vi "high pass filter.vi"() -> ()   [LabVIEW 2010]
uses:
  <vilib>/Utility/file.llb/Write To Spreadsheet File (I64).vi
panel:
  out "x-y":u16=178
  out "Current Aquisiton":u16[](graph)=[1897, 1897, 1897, 1893, 1891, 1889, 1889, 1886, 1885, 1882, 1880, 1875, 1870, 1866, 1863, 1859, 1857, 1852, 1848, 1844, 1839, 1835, 1832, 1829, 1827, 1825, 1821, 1811, 1806, 1801, 1798, 1795, 1794, 1791, 1788, 1786, 1781, 1776, 1771, 1768, 1764, 1762, 1758, 1755, 1751, 1746, 1744, 1742, 1740, 1737, 1737, 1735, 1734, 1733, 1730, 1727, 1728, 1726, 1727, 1726, 1727, 1727, 1726, 1725, 1723, 1728, 1728, 1730, 1730, 1731, 1731, 1732, 1733, 1736, 1738, 1741, 1744, 1745, 1749, 1750, 1752, 1755, 1760, 1764, 1769, 1773, 1776, 1779, 1782, 1786, 1788, 1793, 1797, 1813, 1822, 1826, 1830, 1833, 1837, 1841, 1846, 1850, 1855, 1857, 1861, 1864, 1867, 1871, 1876, 1877, 1882, 1884, 1886, 1888, 1889, 1892, 1893, 1894, 1897, 1898, 1897, 1897, 1897, 1899, 1898, 1900, 1900, 1900, 1898, 1897, 1896, 1895, 1897, 1896, 1894, 1894, 1892, 1889, 1885, 1883, 1880, 1878, 1874, 1873, 1869, 1864, 1858, 1854, 1850, 1846, 1843, 1840, 1837, 1833, 1829, 1826, 1824, 1818, 1810, 1806, 1803, 1800, 1797, 1793, 1790, 1786, 1783, 1781, 1777, 1772, 1769, 1764, 1759, 1757, 1754, 1751, 1749, 1748, 1742, 1740, 1737, 1733, 1733, 1734, 1732, 1731, 1729, 1729, 1726, 1726, 1725, 1726, 1726, 1726, 1728, 1727, 1729, 1726, 1727, 1729, 1733, 1732, 1734, 1736, 1736, 1737, 1739, 1740, 1746, 1749, 1752, 1755, 1758, 1760, 1764, 1767, 1772, 1777, 1781, 1785, 1787, 1789, 1792, 1796, 1813, 1822, 1828, 1832, 1834, 1838, 1841, 1845, 1850, 1854, 1859, 1864, 1866, 1869, 1872, 1874, 1876, 1881, 1886, 1888, 1890, 1890, 1893, 1892, 1895, 1896, 1897, 1899, 1900, 1899, 1898, 1897, 1898, 1899, 1898, 1898, 1900, 1899, 1896, 1894, 1894, 1893, 1891, 1890, 1890, 1887, 1884, 1880, 1877, 1872, 1870, 1867, 1865, 1859, 1855, 1850, 1846, 1842, 1838, 1835, 1834, 1830, 1827, 1824, 1816, 1808, 1804, 1802, 1800, 1797, 1794, 1790, 1786, 1781, 1778, 1775, 1773, 1769, 1766, 1761, 1757, 1753, 1750, 1746, 1745, 1743, 1742, 1738, 1736, 1732, 1730, 1730, 1731, 1729, 1729, 1727, 1726, 1727, 1725, 1726, 1726, 1728, 1730, 1728, 1727, 1728, 1729, 1730, 1732, 1736, 1736, 1736, 1737, 1740, 1741, 1744, 1748, 1751, 1754, 1759, 1761, 1764, 1768, 1772, 1777, 1781, 1786, 1789, 1791, 1793, 1798, 1814, 1822, 1827, 1833, 1836, 1839, 1842, 1846, 1850, 1854, 1858, 1862, 1867, 1869, 1873, 1875, 1877, 1882, 1885, 1888, 1889, 1892, 1891, 1894, 1893, 1896, 1897, 1899, 1899, 1899, 1899, 1898, 1898, 1897, 1898, 1899, 1898, 1899, 1897, 1896, 1894, 1893, 1893, 1892, 1890, 1886, 1883, 1880, 1877, 1872, 1870, 1867, 1863, 1861, 1855, 1850, 1845, 1841, 1838, 1836, 1832, 1830, 1826, 1824, 1814, 1807, 1804, 1802, 1799, 1797, 1794, 1790, 1785, 1781, 1778, 1775, 1773, 1769, 1765, 1760, 1754, 1750, 1750, 1746, 1746, 1742, 1741, 1738, 1733, 1733, 1733, 1731, 1730, 1731, 1730, 1726, 1725, 1726, 1726, 1726, 1727, 1728, 1728, 1729, 1727, 1728, 1728, 1730, 1733, 1734, 1736, 1736, 1738, 1739, 1742, 1746, 1748, 1752, 1756, 1759, 1762, 1765, 1768, 1773, 1777, 1782, 1785, 1788, 1791, 1793, 1801, 1815, 1824, 1829, 1833, 1837, 1839, 1842, 1846, 1850, 1854, 1860, 1864, 1867, 1870, 1872, 1875, 1877, 1881, 1885, 1888, 1889, 1891, 1891, 1893, 1895, 1897, 1898, 1900, 1901, 1898, 1897, 1896, 1898, 1899, 1899, 1900, 1898, 1896, 1897, 1895, 1893, 1893, 1892, 1890, 1889, 1886, 1882, 1880, 1876, 1873, 1870, 1867, 1864, 1859, 1854, 1849, 1844, 1841, 1838, 1835, 1833, 1829, 1826, 1823, 1814, 1807, 1803, 1801, 1799, 1796, 1794, 1789, 1785, 1781, 1778, 1776, 1772, 1768, 1764, 1759, 1756, 1753, 1749, 1747, 1745, 1743, 1741, 1736, 1734, 1733, 1731, 1731, 1730, 1729, 1727, 1728, 1726, 1724, 1726, 1726, 1728, 1728, 1727, 1729, 1729, 1728, 1728, 1730, 1734, 1733, 1736, 1737, 1738, 1741, 1743, 1745, 1749, 1753, 1757, 1759, 1762, 1764, 1769, 1774, 1778, 1782, 1786, 1789, 1791, 1793, 1803, 1817, 1824, 1830, 1833, 1836, 1839, 1842, 1845, 1851, 1855, 1860, 1864, 1867, 1871, 1872, 1875, 1880, 1882, 1886, 1887, 1888, 1891, 1891, 1892, 1894, 1895, 1897, 1899, 1899, 1899, 1897, 1898, 1897, 1898, 1897, 1899, 1898, 1897, 1894, 1895, 1892, 1891, 1893, 1890, 1890, 1887, 1882, 1879, 1874, 1872, 1869, 1866, 1863, 1859, 1854, 1849, 1844, 1841, 1837, 1834, 1832, 1829, 1826, 1823, 1813, 1806, 1802, 1801, 1798, 1797, 1792, 1788, 1785, 1780, 1777, 1774, 1771, 1769, 1763, 1759, 1755, 1750, 1748, 1745, 1746, 1742, 1741, 1739, 1734, 1734, 1731, 1730, 1731, 1731, 1728, 1726, 1726, 1727, 1725, 1726, 1726, 1727, 1730, 1729, 1730, 1728, 1730, 1730, 1733, 1735, 1736, 1739, 1740, 1740, 1742, 1745, 1747, 1754, 1758, 1761, 1763, 1766, 1769, 1772, 1778, 1782, 1786, 1789, 1792, 1794, 1805, 1817, 1824, 1829, 1834, 1838, 1841, 1843, 1846, 1851, 1855, 1859, 1865, 1868, 1871, 1874, 1876, 1880, 1881, 1886, 1888, 1890, 1891, 1893, 1893, 1894, 1896, 1896, 1897, 1899, 1899, 1899, 1897, 1897, 1898, 1901, 1899, 1900, 1898, 1897, 1895, 1894, 1892, 1890, 1890, 1889, 1886, 1882, 1880, 1875, 1871, 1867, 1865, 1862, 1858, 1853, 1849, 1844, 1840, 1837, 1834, 1832, 1829, 1826, 1824, 1812, 1806, 1802, 1800, 1798, 1796, 1793, 1789, 1784, 1781, 1777, 1774, 1771, 1767, 1763, 1760, 1755, 1751, 1746, 1746, 1744, 1742, 1740, 1740, 1736, 1732, 1730, 1730, 1730, 1730, 1729, 1730, 1727, 1726, 1726, 1725, 1727, 1728, 1728, 1730, 1730, 1728, 1730, 1730, 1733, 1735, 1737, 1739, 1739, 1741, 1743, 1745, 1750, 1752, 1757, 1760, 1764, 1766, 1770, 1774, 1778, 1782, 1787, 1790, 1793, 1795, 1807, 1818, 1824, 1829, 1833, 1838, 1842, 1845, 1848, 1851, 1855, 1860, 1864, 1870, 1873, 1876, 1877, 1879, 1882, 1884, 1888, 1892, 1893, 1893, 1893, 1894, 1895, 1897, 1897, 1899, 1900, 1900, 1898, 1899, 1898, 1896, 1897, 1898, 1898, 1898, 1896, 1894, 1891, 1890, 1888, 1889, 1886, 1884, 1880, 1876, 1870, 1867, 1863, 1860, 1857, 1854, 1848, 1845, 1840, 1835, 1833, 1830, 1828, 1826, 1823, 1813, 1806, 1801, 1799, 1797, 1795, 1792, 1789, 1786, 1781, 1776, 1773, 1769, 1766, 1763, 1759, 1757, 1751, 1748, 1743, 1742, 1741, 1741, 1738, 1736, 1734, 1731, 1730, 1730, 1727, 1729, 1729, 1728, 1726, 1728, 1725, 1725, 1726, 1730, 1728, 1730, 1731, 1730, 1730, 1731, 1734, 1736, 1738, 1742, 1743, 1744, 1746, 1749, 1753, 1756, 1761, 1765]
  in  "Auto Save Data":bool=TRUE
  in  "Data File path Ending":string=".dat"
  out "Previous Aquisition":u16[](graph)=[1899, 1898, 1899, 1897, 1897, 1897, 1899, 1900, 1898, 1900, 1898, 1897, 1900, 1898, 1898, 1898, 1897, 1898, 1900, 1898, 1901, 1896, 1899, 1899, 1896, 1899, 1900, 1897, 1901, 1898, 1897, 1898, 1897, 1899, 1900, 1896, 1898, 1897, 1899, 1898, 1897, 1899, 1899, 1898, 1900, 1897, 1899, 1898, 1897, 1899, 1899, 1897, 1899, 1898, 1899, 1899, 1896, 1899, 1897, 1898, 1900, 1898, 1899, 1896, 1898, 1898, 1898, 1897, 1899, 1898, 1900, 1898, 1897, 1899, 1897, 1898, 1899, 1897, 1899, 1898, 1898, 1899, 1898, 1898, 1898, 1897, 1897, 1898, 1899, 1899, 1897, 1901, 1898, 1898, 1900, 1897, 1899, 1900, 1896, 1898, 1898, 1898, 1900, 1898, 1898, 1901, 1896, 1899, 1899, 1897, 1900, 1897, 1898, 1899, 1897, 1899, 1897, 1897, 1900, 1897, 1899, 1899, 1897, 1900, 1898, 1898, 1898, 1897, 1898, 1899, 1897, 1899, 1898, 1897, 1899, 1895, 1900, 1900, 1899, 1900, 1897, 1897, 1899, 1896, 1898, 1898, 1896, 1898, 1897, 1897, 1898, 1896, 1898, 1898, 1898, 1899, 1896, 1898, 1898, 1897, 1898, 1897, 1899, 1901, 1898, 1898, 1899, 1896, 1900, 1898, 1897, 1900, 1899, 1897, 1900, 1898, 1900, 1898, 1899, 1900, 1898, 1900, 1899, 1898, 1898, 1897, 1898, 1899, 1897, 1900, 1898, 1897, 1900, 1897, 1897, 1898, 1896, 1899, 1898, 1897, 1901, 1897, 1898, 1900, 1898, 1898, 1899, 1898, 1901, 1896, 1898, 1898, 1897, 1901, 1898, 1898, 1898, 1898, 1898, 1898, 1897, 1900, 1898, 1898, 1899, 1897, 1899, 1898, 1897, 1898, 1899, 1898, 1899, 1897, 1899, 1898, 1898, 1898, 1897, 1898, 1899, 1897, 1899, 1899, 1900, 1900, 1897, 1899, 1898, 1898, 1899, 1899, 1898, 1899, 1898, 1899, 1900, 1897, 1900, 1898, 1898, 1899, 1896, 1899, 1899, 1897, 1899, 1897, 1898, 1899, 1898, 1898, 1898, 1899, 1899, 1896, 1897, 1899, 1897, 1900, 1899, 1899, 1899, 1897, 1898, 1899, 1897, 1899, 1898, 1898, 1900, 1896, 1899, 1898, 1898, 1900, 1898, 1899, 1900, 1897, 1899, 1898, 1898, 1898, 1899, 1898, 1900, 1898, 1900, 1899, 1897, 1899, 1897, 1900, 1899, 1897, 1899, 1898, 1897, 1900, 1897, 1897, 1898, 1896, 1900, 1899, 1899, 1901, 1898, 1899, 1900, 1897, 1899, 1898, 1898, 1899, 1898, 1899, 1900, 1897, 1900, 1897, 1897, 1899, 1897, 1900, 1899, 1896, 1900, 1897, 1898, 1900, 1896, 1898, 1898, 1897, 1899, 1896, 1898, 1900, 1896, 1900, 1899, 1897, 1901, 1899, 1899, 1899, 1899, 1899, 1898, 1897, 1900, 1898, 1899, 1899, 1897, 1900, 1898, 1898, 1898, 1896, 1898, 1900, 1897, 1898, 1898, 1898, 1901, 1896, 1900, 1898, 1898, 1899, 1898, 1898, 1898, 1898, 1898, 1898, 1897, 1899, 1897, 1897, 1899, 1898, 1899, 1897, 1897, 1898, 1896, 1899, 1899, 1897, 1899, 1898, 1897, 1901, 1897, 1899, 1898, 1897, 1899, 1898, 1896, 1899, 1896, 1898, 1898, 1896, 1899, 1897, 1899, 1899, 1898, 1897, 1899, 1896, 1899, 1897, 1898, 1898, 1897, 1900, 1898, 1897, 1898, 1898, 1899, 1898, 1897, 1899, 1897, 1898, 1897, 1899, 1898, 1897, 1896, 1899, 1899, 1897, 1899, 1897, 1898, 1897, 1897, 1899, 1897, 1898, 1900, 1894, 1899, 1898, 1898, 1898, 1897, 1899, 1899, 1897, 1898, 1898, 1899, 1899, 1897, 1898, 1898, 1897, 1899, 1898, 1896, 1898, 1897, 1898, 1900, 1898, 1898, 1898, 1897, 1898, 1896, 1898, 1898, 1896, 1900, 1897, 1898, 1900, 1897, 1899, 1899, 1899, 1899, 1895, 1898, 1898, 1897, 1898, 1897, 1898, 1898, 1895, 1897, 1898, 1897, 1897, 1897, 1897, 1899, 1895, 1897, 1897, 1897, 1899, 1898, 1897, 1900, 1896, 1898, 1898, 1896, 1899, 1898, 1896, 1898, 1897, 1898, 1897, 1897, 1899, 1896, 1898, 1898, 1896, 1897, 1897, 1897, 1899, 1896, 1897, 1898, 1896, 1898, 1897, 1897, 1898, 1897, 1898, 1897, 1897, 1898, 1898, 1898, 1898, 1896, 1897, 1897, 1896, 1899, 1897, 1897, 1898, 1896, 1899, 1897, 1896, 1899, 1898, 1896, 1897, 1897, 1897, 1896, 1896, 1900, 1896, 1898, 1898, 1896, 1899, 1896, 1897, 1899, 1895, 1899, 1898, 1896, 1898, 1898, 1895, 1899, 1896, 1898, 1897, 1894, 1897, 1897, 1895, 1898, 1896, 1896, 1899, 1896, 1898, 1898, 1897, 1898, 1899, 1897, 1896, 1896, 1898, 1897, 1897, 1898, 1897, 1899, 1896, 1896, 1898, 1896, 1897, 1897, 1897, 1898, 1896, 1896, 1898, 1896, 1897, 1898, 1897, 1897, 1896, 1897, 1898, 1896, 1897, 1897, 1896, 1899, 1896, 1896, 1898, 1895, 1898, 1897, 1893, 1898, 1895, 1897, 1897, 1894, 1898, 1896, 1896, 1896, 1895, 1897, 1897, 1896, 1898, 1896, 1895, 1897, 1894, 1897, 1898, 1896, 1897, 1897, 1896, 1897, 1897, 1898, 1896, 1897, 1897, 1896, 1897, 1897, 1895, 1897, 1897, 1897, 1897, 1896, 1896, 1897, 1896, 1897, 1898, 1896, 1897, 1895, 1897, 1897, 1894, 1896, 1897, 1896, 1896, 1894, 1896, 1897, 1894, 1897, 1896, 1896, 1897, 1896, 1896, 1895, 1895, 1897, 1897, 1895, 1897, 1896, 1897, 1897, 1895, 1897, 1896, 1896, 1897, 1895, 1897, 1897, 1895, 1897, 1895, 1896, 1894, 1894, 1896, 1897, 1894, 1897, 1893, 1895, 1898, 1894, 1896, 1894, 1894, 1897, 1895, 1897, 1898, 1894, 1897, 1897, 1894, 1897, 1895, 1894, 1895, 1895, 1897, 1896, 1896, 1897, 1894, 1897, 1897, 1894, 1898, 1894, 1896, 1897, 1893, 1897, 1897, 1894, 1898, 1895, 1894, 1897, 1895, 1897, 1895, 1893, 1897, 1894, 1895, 1896, 1895, 1897, 1895, 1895, 1897, 1895, 1895, 1897, 1895, 1897, 1894, 1895, 1895, 1893, 1896, 1894, 1894, 1897, 1894, 1894, 1896, 1893, 1897, 1897, 1894, 1897, 1894, 1895, 1896, 1895, 1896, 1896, 1893, 1897, 1894, 1895, 1896, 1893, 1897, 1893, 1894, 1897, 1894, 1895, 1895, 1892, 1895, 1894, 1893, 1896, 1894, 1895, 1896, 1894, 1894, 1896, 1894, 1895, 1894, 1894, 1894, 1894, 1895, 1894, 1896, 1895, 1893, 1895, 1895, 1893, 1895, 1894, 1894, 1896, 1894, 1896, 1894, 1894, 1895, 1894, 1893, 1896, 1893, 1895, 1894, 1894, 1894, 1894, 1895, 1895, 1893, 1895, 1893, 1894, 1895, 1894, 1896, 1895, 1893, 1894, 1894, 1895, 1894, 1893, 1895, 1895, 1892, 1895, 1891, 1895, 1896, 1891, 1896, 1893, 1893, 1896, 1893, 1894, 1893, 1894, 1894, 1894, 1894, 1894, 1892, 1895, 1894, 1893, 1895, 1893, 1893, 1896, 1893, 1895, 1894, 1891, 1895, 1892, 1893, 1895, 1892, 1894, 1894, 1894, 1894, 1894, 1893, 1894, 1893, 1893, 1894, 1891, 1893, 1893, 1894, 1895, 1892, 1895, 1895, 1894, 1896, 1891, 1894, 1894, 1894, 1893, 1894, 1893, 1894, 1893, 1894, 1893, 1891, 1893, 1892, 1893, 1894, 1892, 1893, 1892, 1892, 1893, 1892, 1893, 1894, 1891, 1894, 1893, 1892, 1893, 1891, 1893, 1893]
  in  "time format string (%c)":string="%Y-%m-%d %H-%M.%S"
  out "date/time string":string="2012-02-22 16-27.20"
  in  "InterChannel Delay":sgl=-1.0 format="%.2f"
  out "ErrMsg":string="No error has occurred"
  out "ErrCode":i32
  in  "BoardNum":u32
  in  "LowChan":i32
  in  "HighChan":i32
  in  "Options":i32
  in  "Range":i32(ring)=1 items=["Not Programmable"=0, "+- 20 V"=27, "+- 10 V"=1, "+- 5 V"=2, "+- 4 V"=28, "+- 2.5 V"=3, "+- 2 V"=29, "+- 1.67 V"=4, "+- 1.25 V"=5, "+- 1 V"=6, "+- .625 V"=7, "+- .5 V"=8, "+- .25 V"=30, "+- .2 V"=31, "+- .1 V"=9, "+- .05 V"=10, "+- .01 V"=11, "+- .005 V"=12, "0 - 10 V"=13, "0 - 5 V"=14, "0 - 4 V"=36, "0 - 2.5 V"=15, "0 - 2 V"=16, "0 - 1.67 V"=17, "0 - 1.25 V"=18, "0 - 1 V"=19, "0 - .5 V"=32, "0 - .25 V"=33, "0 - .2 V"=34, "0 - .1 V"=20, "0 - .02 V"=35, "0 - .01 V"=21, "4 - 20 mA"=22, "2 - 10 mA"=23, "1 - 5 mA"=24, ".5 - 2.5 mA"=25, "0 - 20 mA"=26]
  in  "Rate":i32=100
  in  "Count":i32=1000
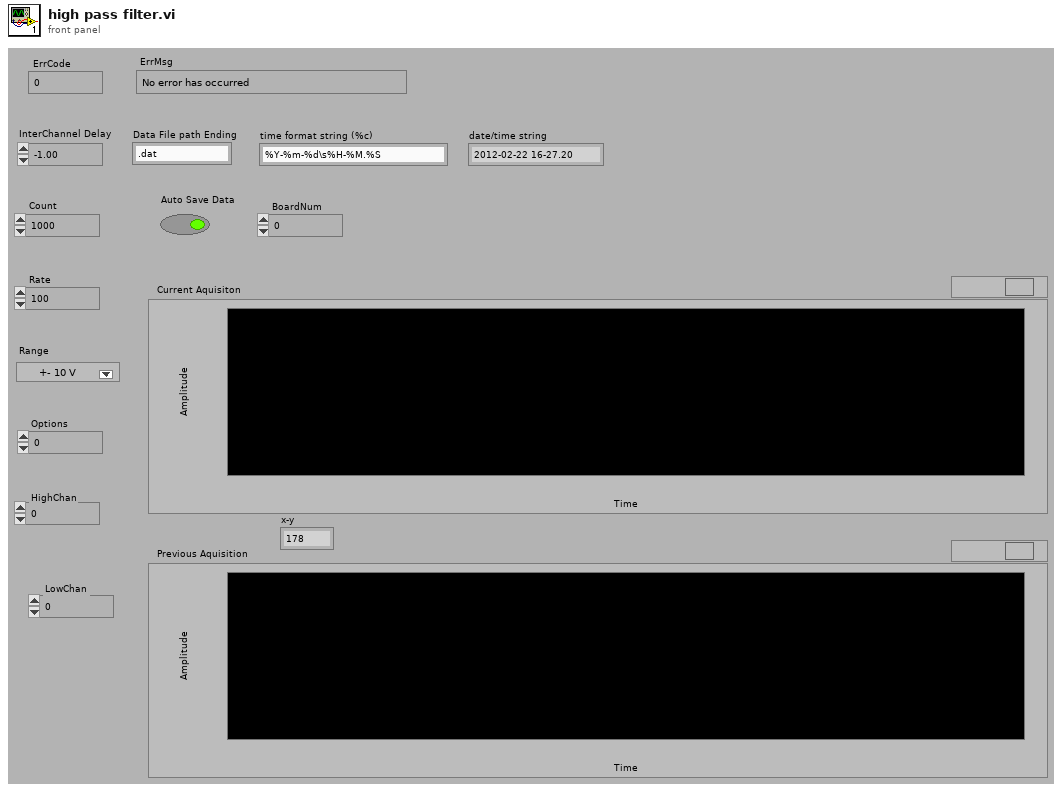
[diagram p1: front panel]
types:
  T1 = typedef "imagedata.ctl" = cluster{"image type":i32, "image depth":i32, "image":u8[], "mask":u8[], "colors":u32[], "Rectangle":cluster{"left":i16, "top":i16, "right":i16, "bottom":i16}}
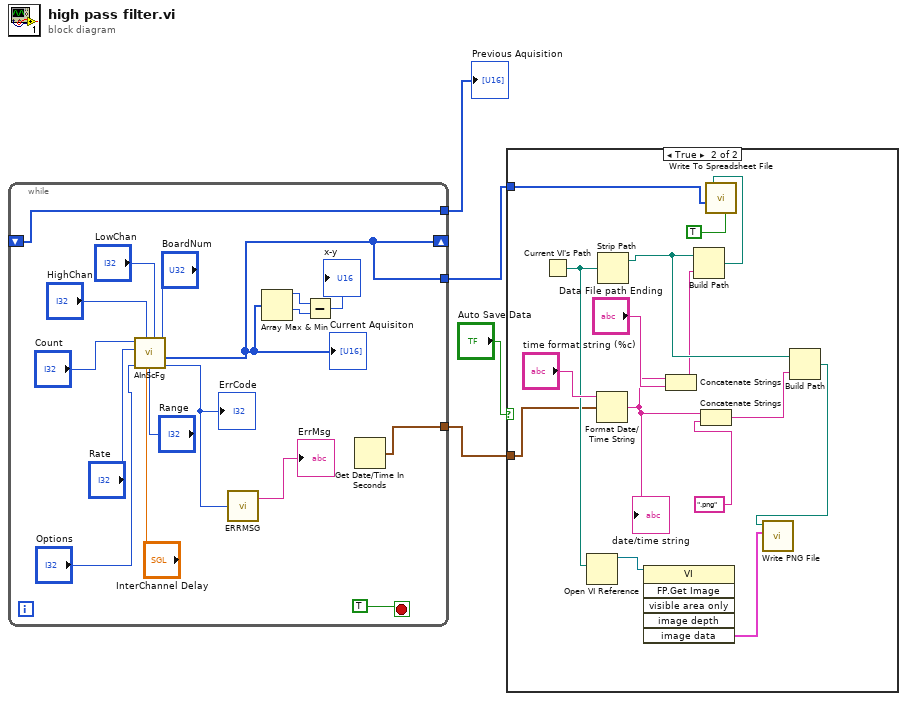
[diagram p0: block diagram]
diagram:
  n1 = while {
    shift-right: [w8] -> _
    shift-left: _ -> [w11]
    tunnel: [w11] -> w4
    tunnel: [w8] -> w3
    tunnel: [w9] -> w2
    stop <- TRUE stop-if-true
    n2 = call <menus>:"AInScFg.VI"("BoardNum"="BoardNum", "LowChan"="LowChan", "InterChannel Delay"="InterChannel Delay", "HighChan"="HighChan", "Options"="Options", "Range"="Range", "Rate"="Rate", "Count"="Count") -> ("ErrCode"=w14:i32, "ADData"=w8:u16[])  [unwired: 1 out]
    "ErrCode" <- w14
    "Current Aquisiton" <- w8
    n3 = call <menus>:"ERRMSG.VI"("ErrCode"=w14) -> ("ErrMsg"=→"ErrMsg":string)  [unwired: 1 out]
    n4 = Array Max & Min(array=w8) -> (max value=w7:u16, min value=w6:u16)  [unwired: 2 out]
    n5 = Subtract(x=w7, y=w6) -> (x-y=→"x-y":u16)
    n6 = Get Date/Time In Seconds() -> (seconds since 1Jan1904=w9:timestamp)
  }
  "Previous Aquisition" <- w4
  n7 = case shown="True" "Auto Save Data" {
    tunnel: w3 -> [_ w30]
    tunnel: w2 -> [_ w27]
    frame False {
    }
    frame True {
      n8 = Current VI's Path() -> (path=w29:path)
      n9 = Open VI Reference(vi path=w29) -> (vi reference=w25:refnum<vi>)  [unwired: 5 in, 1 out]
      n10 = Format Date/Time String(time format string (%c)="time format string (%c)", seconds (now)=w27) -> (date/time string=w22:string)  [unwired: 1 in]
      "date/time string" <- w22
      n11 = Strip Path(path=w29) -> (stripped path=w36:path)  [unwired: 1 out]
      n12 = invoke class="VI" method="FP.Get Image"(reference=w25) -> ("image data"=w26:T1)  [unwired: 5 in, 5 out]
      n13 = Concatenate Strings(w22, "Data File path Ending") -> (w23:string)
      n14 = Build Path(base path=w36, name or relative path=w23) -> (appended path=w24:path)
      n15 = Concatenate Strings(w22, ".png") -> (w35:string)
      n16 = call-poly <vilib>:"Write To Spreadsheet File.vi"("transpose? (no:F)"=TRUE, "1D data"=w30, "file path (dialog if empty)"=w24) -> ()  [unwired: 5 in, 1 out]
      n17 = Build Path(base path=w36, name or relative path=w35) -> (appended path=w34:path)
      n18 = call <vilib>:"Write PNG File.vi"("image data"=w26, "path to PNG file"=w34) -> ()  [unwired: 8 in, 2 out]
    }
  }
